vi "coords_ROI_currentimage.vi"() -> (0 "Mono ROI":i32[](array[numeric]))   [LabVIEW 2019]
uses:
  red_tweezers_globals_INTERNAL.vi
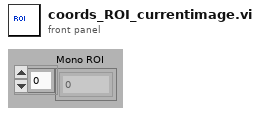
[diagram p1: front panel]
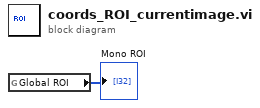
[diagram p0: block diagram]
diagram:
  n1 = global read "red_tweezers_globals_INTERNAL.vi" "Global ROI"() -> (→"Mono ROI":i32[])
